vi "default file paths.vi"() -> (2 "paths":T1)   [LabVIEW 2014, in "Standard Editor.lvlib"]
doc: "Get default file paths to cache, glyph, and INI files used within the DCAF editor."
uses:
  Standard Editor.lvlib
  Controls/FilePaths.ctl
  <vilib>/Utility/libraryn.llb/Check if File or Folder Exists.vi
  Framework Configuration Classes/class cache/PL_class cache.lvlib
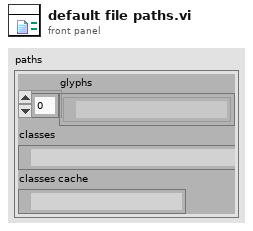
[diagram p1: front panel]
types:
  T1 = typedef "Standard Editor.lvlib/FilePaths.ctl" = cluster{"glyphs":path[], "classes":path, "classes cache":path}
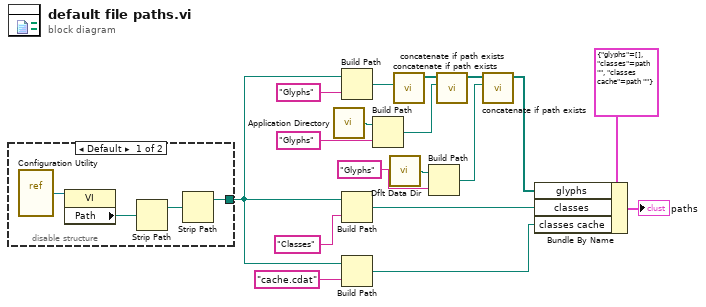
[diagram p0: block diagram]
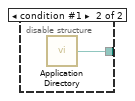
[diagram p2: hidden frame]
diagram:
  n1 = disable-structure shown="Default" {
    disable-tunnel: [w20 w23] -> w1
    frame condition #0 (active) {
      n2 = vi-ref "Configuration Utility.vi"() -> (w22:refnum<vi>)
      n3 = property class="VI"(reference=w22) -> ("Path"=w21:path)  [unwired: 1 in, 2 out]
      n4 = Strip Path(path=w21) -> (stripped path=w19:path)  [unwired: 1 out]
      n5 = Strip Path(path=w19) -> (stripped path=w20:path)  [unwired: 1 out]
    }
    frame condition #1 {
      n6 = call <vilib>:"Application Directory.vi"() -> ("Application Directory"=w23:path)
    }
  }
  n7 = call <vilib>:"Application Directory.vi"() -> ("Application Directory"=w13:path)
  n8 = Build Path(base path=w1, name or relative path="Glyphs") -> (appended path=w3:path)
  n9 = Build Path(base path=w1, name or relative path="Classes") -> (appended path=w14:path)
  n10 = Build Path(base path=w1, name or relative path="cache.cdat") -> (appended path=w2:path)
  n11 = Build Path(base path=w13, name or relative path="Glyphs") -> (appended path=w8:path)
  n12 = call <vilib>:"Dflt Data Dir.vi"() -> ("App:Default Data Directory"=w10:path)
  n13 = call "concatenate if path exists.vi"("new path"=w3) -> ("paths out"=w4:path[])  [unwired: 10 in]
  n14 = Build Path(base path=w10, name or relative path="Glyphs") -> (appended path=w9:path)
  n15 = call "concatenate if path exists.vi"("new path"=w8, "paths in"=w4) -> ("paths out"=w7:path[])  [unwired: 9 in]
  n16 = call "concatenate if path exists.vi"("new path"=w9, "paths in"=w7) -> ("paths out"=w6:path[])  [unwired: 9 in]
  n17 = Bundle By Name(cluster=T1 {"glyphs"=[], "classes"=path "", "classes cache"=path ""} ("Cluster 2"), "glyphs"=w6, "classes"=w14, "classes cache"=w2) -> (→"paths":T1)
